vi "Configure Measurements (Standby).vi"(8 "error in (no error)":errorcluster, 9 "Averaging Period (10sec)":i32=10 min=1 max=300 step=1, 10 "Standby Measurements":i32[](listbox)=[0, 1, 2, 5, 6, 7, 8], 11 "VISA resource name":refnum<visa-resource-name>) -> (0 "error out":errorcluster, 3 "VISA resource name out":refnum<visa-resource-name>)   [LabVIEW 2015, in "Voltech PM1000+.lvlib"]
doc: "Configures the measurement itmes, and return the selected measurement list and indicators. This vi is used when PM1000+ is set to Standby mode by using \"Configure Mode\" vi."
uses:
  <instrlib>/Voltech PM1000+/Voltech PM1000+.lvlib
panel:
  # "Notice:  \nHold \"Ctrl\" key and click the \nmeasurements to select \nmultiple items."
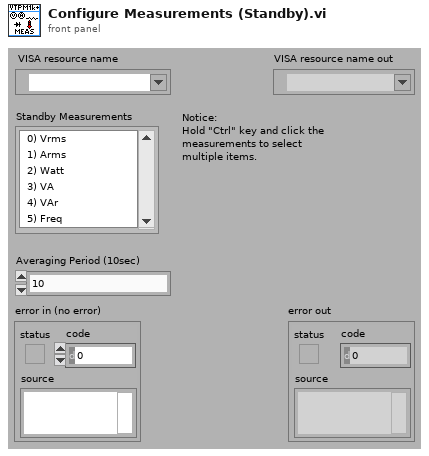
[diagram p1: front panel]
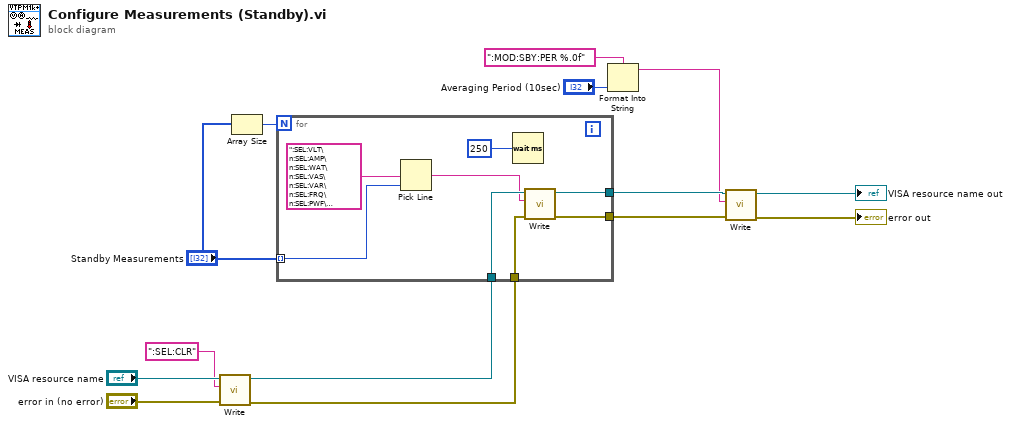
[diagram p0: block diagram]
diagram:
  n1 = call <instrlib>:"Write.vi"("error in (no error)"="error in (no error)", "Write Buffer"=":SEL:CLR" ("multi-line string"), "VISA resource name"="VISA resource name") -> ("error out"=w7:errorcluster, "VISA resource name out"=w8:refnum<visa-resource-name>)  [unwired: 7 in]
  n2 = Array Size(array="Standby Measurements") -> (size(s)=w12:i32)
  n3 = for {
    N: w12 -> [_]
    tunnel: "Standby Measurements" -> [w21] mode=indexing
    tunnel: w8 -> [w20]
    tunnel: w7 -> [w19]
    tunnel: [w18] -> w6
    tunnel: [w17] -> w5
    n4 = Pick Line(multi-line string=":SEL:VLT\n:SEL:AMP\n:SEL:WAT\n:SEL:VAS\n:SEL:VAR\n:SEL:FRQ\n:SEL:PWF\n:SEL:VPK+\n:SEL:VPK-\n:SEL:APK+\n:SEL:APK-\n:SEL:VDC\n:SEL:ADC\n:SEL:VCF\n:SEL:ACF\n:SEL:VDF\n:SEL:ADF\n:SEL:IMP\n:SEL:RES\n:SEL:REA\n:SEL:VHM\n:SEL:AHM\n:SEL:VRNG\n:SEL:ARNG", line index=w21) -> (output string=w15:string)  [unwired: 1 in]
    n5 = Wait (ms)(milliseconds to wait=250) -> ()  [unwired: 1 out]
    n6 = call <instrlib>:"Write.vi"("error in (no error)"=w19, "Write Buffer"=w15, "VISA resource name"=w20) -> ("error out"=w17:errorcluster, "VISA resource name out"=w18:refnum<visa-resource-name>)  [unwired: 7 in]
  }
  n7 = Format Into String(format string=":MOD:SBY:PER %.0f", "Averaging Period (10sec)") -> (resulting string=w3:string)  [unwired: 2 in, 1 out]
  n8 = call <instrlib>:"Write.vi"("error in (no error)"=w5, "Write Buffer"=w3, "VISA resource name"=w6) -> ("error out"=→"error out":errorcluster, "VISA resource name out"=→"VISA resource name out":refnum<visa-resource-name>)  [unwired: 7 in]
